vi "prepare_lookup.vi"(7 "progress bar ref":refnum<vi>, 8 "error in (no error)":errorcluster, 11 "PositionSignals in":refnum<class "PositionSignals.lvclass">) -> (0 "error out":errorcluster, 3 "PositionSignals out":refnum<class "PositionSignals.lvclass">)   [LabVIEW 2010, in "PositionSignals.lvclass"]
uses:
  PositionSignals.lvclass
  common/classes/Image/Image/position_channels_cluster.ctl
  common/classes/Image/Image/Image.lvclass
  PositionSignals.lvclass/PositionSignals.ctl
  common/classes/ImageCollection/ImageCollection/ImageCollection.lvclass
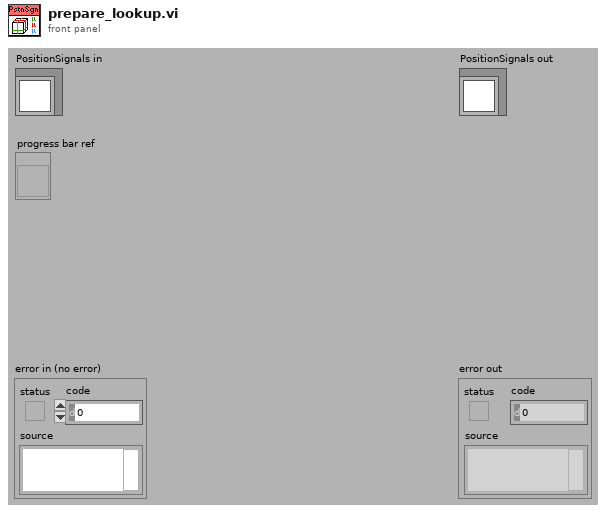
[diagram p1: front panel]
types:
  T1 = typedef "Image.lvclass/position_channels_cluster.ctl" = cluster{"x":refnum<class "Image.lvclass">, "y":refnum<class "Image.lvclass">, "z":refnum<class "Image.lvclass">}
  T2 = cluster{"x/y/z coordinates[0]":refnum<class "ImageCollection.lvclass">, "x/y/z coordinates[1]":refnum<class "ImageCollection.lvclass">, "x/y/z coordinates[2]":refnum<class "ImageCollection.lvclass">}
  T3 = typedef "Image.lvclass/pixel_positions_cluster.ctl" = cluster{"x":dbl[], "y":dbl[], "z":dbl}
  T4 = cluster{"[0]":cluster{"mean values":dbl[]}, "[1]":cluster{"mean values":dbl[]}}
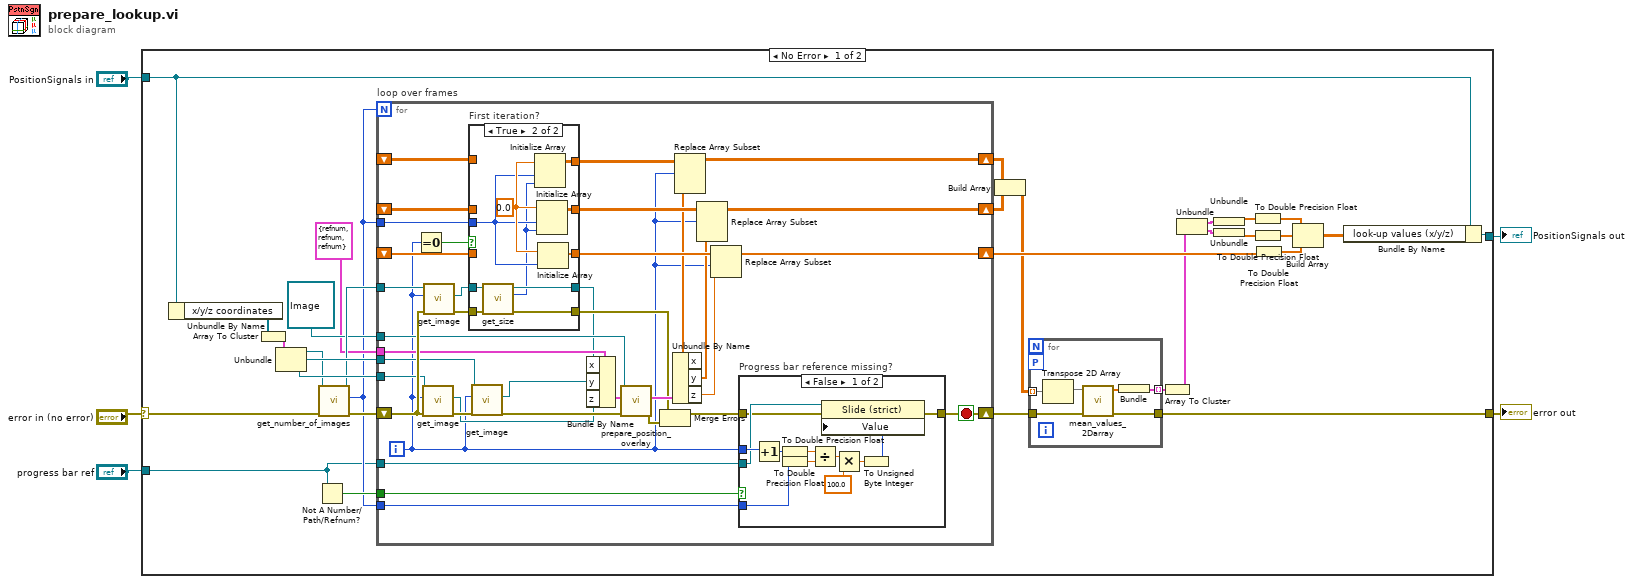
[diagram p0: block diagram]
diagram:
  n1 = case shown="No Error" "error in (no error)" {
    selector: "error in (no error)" -> [w10 w109]
    tunnel: [w11 w109] -> w2
    tunnel: [w16 w108] -> w1
    tunnel: "PositionSignals in" -> [w13 w108]
    tunnel: "progress bar ref" -> [w15 _]
    frame No Error {
      n2 = Unbundle By Name(w13) -> ("x/y/z coordinates"=w12:refnum<class "ImageCollection.lvclass">[])
      n3 = Array To Cluster(array=w12) -> (cluster=w14:T2)
      n4 = Unbundle(w14) -> ("x/y/z coordinates[0]"=w33:refnum<class "ImageCollection.lvclass">, "x/y/z coordinates[1]"=w36:refnum<class "ImageCollection.lvclass">, "x/y/z coordinates[2]"=w35:refnum<class "ImageCollection.lvclass">)
      n5 = Not A Number/Path/Refnum?(number/path/refnum=w15) -> (NaN/Path/Refnum?=w20:bool)
      n6 = call-dynamic "get_number_of_images.vi"("error in (no error)"=w10, "ImageCollection in"=w33) -> ("error out"=w31:errorcluster, "size"=w19:i32, "ImageCollection out"=w32:refnum<class "ImageCollection.lvclass">)  [unwired: 7 in]
      n7 = for "loop over frames" {
        N: w19 -> [_]
        shift-right: [w78] -> w29
        shift-left: _ -> [w69]
        shift-right: [w79] -> w30
        shift-left: _ -> [w68]
        shift-right: [w77] -> w34
        shift-left: _ -> [w64]
        shift-right: [w43] -> w18
        shift-left: w31 -> [w76]
        tunnel: w32 -> [w75]
        tunnel: w36 -> [w74]
        tunnel: w35 -> [w73]
        tunnel: w19 -> [w71]
        tunnel: refnum<class "Image.lvclass"> refnum ("Image.lvclass") -> [w56]
        tunnel: T1 {"x"=refnum, "y"=refnum, "z"=refnum} ("position channels") -> [w53]
        tunnel: w15 -> [w45]
        tunnel: w20 -> [w44]
        tunnel: w19 -> [w46]
        i -> [w48]
        stop <- w43 stop-if-true
        n8 = Equal To 0?(x=w48) -> (x = 0?=w65:bool)
        n9 = call-dynamic "get_image.vi"("error in (no error)"=w76, "index"=w48, "ImageCollection in"=w73) -> ("error out"=w58:errorcluster, "Image.lvclass"=w51:refnum<class "Image.lvclass">)  [unwired: 6 in, 1 out]
        n10 = call-dynamic "get_image.vi"("error in (no error)"=w76, "index"=w48, "ImageCollection in"=w75) -> ("error out"=w67:errorcluster, "Image.lvclass"=w66:refnum<class "Image.lvclass">)  [unwired: 6 in, 1 out]
        n11 = case "First iteration?" shown="True" w65 {
          tunnel: w67 -> [w94 w107]
          tunnel: w66 -> [w95 w106]
          tunnel: [w97 w105] -> w72
          tunnel: w71 -> [_ w99]
          tunnel: [w96 w104] -> w70
          tunnel: w69 -> [w97 _]
          tunnel: w68 -> [w96 _]
          tunnel: [w94 w103] -> w55
          tunnel: [w95 w102] -> w49
          tunnel: w64 -> [w93 _]
          tunnel: [w93 w100] -> w63
          frame False {
          }
          frame True {
            w101 = 0.0 ("Numeric")
            n12 = call-dynamic "get_size.vi"("error in (no error)"=w107, "Image in"=w106) -> ("error out"=w103:errorcluster, "x resolution"=w98:i32, "Image out"=w102:refnum<class "Image.lvclass">)  [unwired: 2 in, 5 out]
            n13 = Initialize Array(w101, w99, w98) -> (w104:dbl[][])
            n14 = Initialize Array(w101, w99, w98) -> (w105:dbl[][])
            n15 = Initialize Array(w101, w99) -> (w100:dbl[])
          }
        }
        n16 = call-dynamic "get_image.vi"("error in (no error)"=w58, "index"=w48, "ImageCollection in"=w74) -> ("error out"=w57:errorcluster, "Image.lvclass"=w52:refnum<class "Image.lvclass">)  [unwired: 6 in, 1 out]
        n17 = Bundle By Name(cluster=w53, "x"=w49, "y"=w52, "z"=w51) -> (w50:T1)
        n18 = call "prepare_position_overlay.vi"("error in (no error)"=w57, "position channels"=w50, "Image in"=w56) -> ("error out"=w54:errorcluster, "pixel positions"=w62:T3)  [unwired: 6 in, 1 out]
        n19 = Merge Errors(w55, w54) -> (w47:errorcluster)
        n20 = Unbundle By Name(w62) -> ("x"=w61:dbl[], "y"=w60:dbl[], "z"=w59:dbl)
        n21 = Replace Array Subset(array=w70, new element=w61, index (row)=w48) -> (w79:dbl[][])  [unwired: 1 in]
        n22 = Replace Array Subset(array=w72, new element=w60, index (row)=w48) -> (w78:dbl[][])  [unwired: 1 in]
        n23 = Replace Array Subset(array=w63, new element=w59, index=w48) -> (w77:dbl[])
        n24 = case "Progress bar reference missing?" shown="False" w44 {
          tunnel: w46 -> [w87 _]
          tunnel: w48 -> [w84 _]
          tunnel: w45 -> [w83 _]
          tunnel: w47 -> [w82 w92]
          tunnel: [w81 w92] -> w43
          frame False {
            n25 = Increment(x=w84) -> (x+1=w85:i32)
            n26 = To Double Precision Float(number=w85) -> (double precision float=w88:dbl)
            n27 = To Double Precision Float(number=w87) -> (double precision float=w86:dbl)
            n28 = Divide(x=w88, y=w86) -> (x/y=w91:dbl)
            n29 = Multiply(x=w91, y=100.0) -> (x*y=w89:dbl)
            n30 = To Unsigned Byte Integer(number=w89) -> (unsigned 8bit integer=w80:u8)
            n31 = property class="Slide (strict)"(reference=w83, error in=w82, "Value"=w80) -> (error out=w81:errorcluster)  [unwired: 1 out]
          }
          frame True {
          }
        }
      }
      n32 = Build Array(w30, w29) -> (w28:dbl[][][])
      n33 = for {
        tunnel: [w38] -> w27 mode=indexing
        tunnel: w28 -> [w42] mode=indexing
        workers-P: _ -> [_]
        tunnel: w18 -> [w40]
        tunnel: [w37] -> w11
        n34 = Transpose 2D Array(2D array=w42) -> (transposed array=w41:dbl[][])
        n35 = call "mean_values_2Darray.vi"("error in (no error)"=w40, "Array"=w41) -> ("error out"=w37:errorcluster, "mean values"=w39:dbl[])  [unwired: 6 in]
        n36 = Bundle("mean values"=w39) -> (w38:cluster{"mean values":dbl[]})  [unwired: 1 in]
      }
      n37 = Array To Cluster(array=w27) -> (cluster=w17:T4)
      n38 = Unbundle(w17) -> ("[0]"=w26:cluster{"mean values":dbl[]}, "[1]"=w24:cluster{"mean values":dbl[]})
      n39 = Unbundle(w26) -> ("mean values"=w25:dbl[])
      n40 = Unbundle(w24) -> ("mean values"=w23:dbl[])
      n41 = To Double Precision Float(number=w25) -> (double precision float=w9:dbl[])
      n42 = To Double Precision Float(number=w23) -> (double precision float=w7:dbl[])
      n43 = To Double Precision Float(number=w34) -> (double precision float=w8:dbl[])
      n44 = Build Array(w9, w7, w8) -> (w6:dbl[][])
      n45 = Bundle By Name(cluster=w13, "look-up values (x/y/z)"=w6) -> (w16:refnum<class "PositionSignals.lvclass">)
    }
    frame Error {
    }
  }
  "error out" <- w2
  "PositionSignals out" <- w1
